vi "Configure TimersCounters UE9.vi"(0 "Handle In":i32, 1 "Enable Counter0":bool, 2 "Enable Counter1":bool, 5 "Timer Clock Base (0=750k, 1=48M)":i32, 7 "Timer Clock Divisor":i32, 9 "# Timers Enabled":i32, 11 "error in":errorcluster, 12 "TimerModes":u8[](array[numeric])=[0, 0, 0, 0, 0, 0], 13 "TimerValues":dbl[](array[numeric])=[0.0, 0.0, 0.0, 0.0, 0.0, 0.0] format="%.2f") -> (4 "Handle Out":i32, 15 "error out":errorcluster)   [LabVIEW 2021]
panel:
  # "Timer0\n\nTimer1\n\nTimer2\n\nTimer3\n\nTimer4\n\nTimer5"
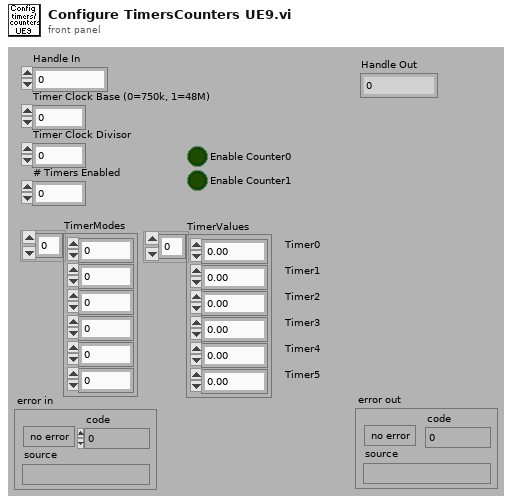
[diagram p1: front panel]
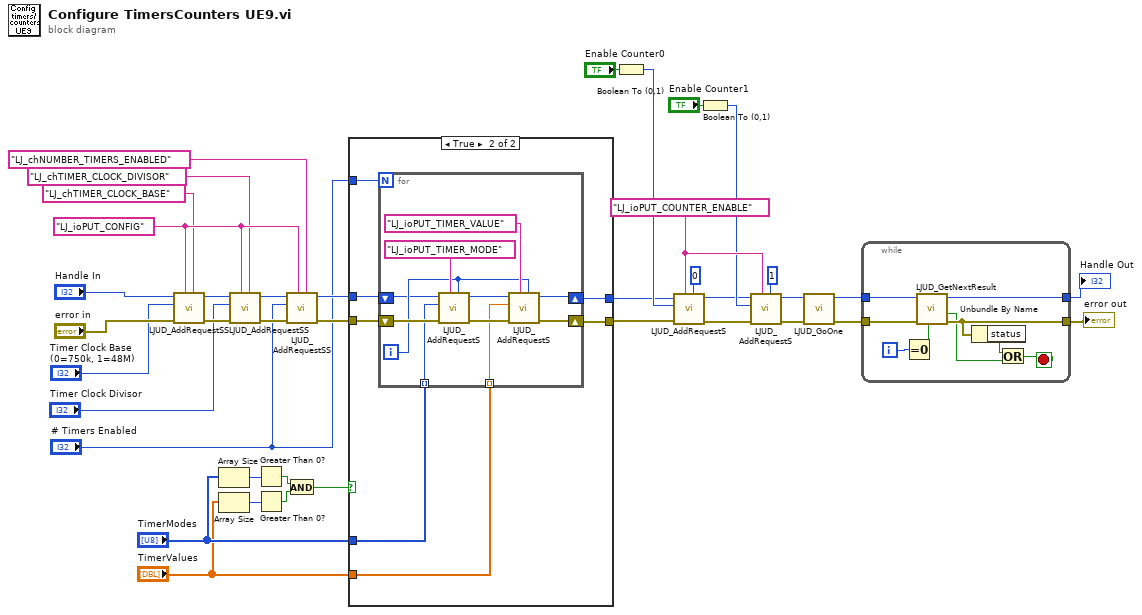
[diagram p0: block diagram]
diagram:
  w17 = "LJ_ioPUT_COUNTER_ENABLE" ("IOType")
  w35 = "LJ_ioPUT_CONFIG" ("IOType")
  n1 = call "LJUD_AddRequestSS.vi"("Channel"="LJ_chTIMER_CLOCK_BASE" ("IOType"), "IOType"=w35, "error in"="error in", "Value"="Timer Clock Base (0=750k, 1=48M)", "Handle In"="Handle In") -> ("error out"=w37:errorcluster, "Handle Out"=w39:i32)  [unwired: 5 in]
  n2 = Array Size(array="TimerModes") -> (size(s)=w22:i32)
  n3 = Array Size(array="TimerValues") -> (size(s)=w21:i32)
  n4 = call "LJUD_AddRequestSS.vi"("Channel"="LJ_chTIMER_CLOCK_DIVISOR" ("IOType"), "IOType"=w35, "error in"=w37, "Value"="Timer Clock Divisor", "Handle In"=w39) -> ("error out"=w36:errorcluster, "Handle Out"=w38:i32)  [unwired: 5 in]
  n5 = Greater Than 0?(x=w22) -> (x > 0?=w19:bool)
  n6 = Greater Than 0?(x=w21) -> (x > 0?=w20:bool)
  n7 = call "LJUD_AddRequestSS.vi"("Channel"="LJ_chNUMBER_TIMERS_ENABLED" ("IOType"), "IOType"=w35, "error in"=w36, "Value"="# Timers Enabled", "Handle In"=w38) -> ("error out"=w25:errorcluster, "Handle Out"=w10:i32)  [unwired: 5 in]
  n8 = And(x=w19, y=w20) -> (x .and. y?=w23:bool)
  n9 = case shown="True" w23 {
    tunnel: w25 -> [w41 w48]
    tunnel: "TimerModes" -> [_ w47]
    tunnel: "TimerValues" -> [_ w46]
    tunnel: [w41 w45] -> w18
    tunnel: w10 -> [w40 w44]
    tunnel: [w40 w43] -> w9
    tunnel: "# Timers Enabled" -> [_ w42]
    frame False {
    }
    frame True {
      n10 = for {
        N: w42 -> [_]
        shift-right: [w51] -> w45
        shift-left: w48 -> [w55]
        tunnel: w47 -> [w54] mode=indexing
        tunnel: w46 -> [w53] mode=indexing
        shift-right: [w49] -> w43
        shift-left: w44 -> [w50]
        i -> [w52]
        n11 = call "LJUD_AddRequestS.vi"("Channel"=w52, "IOType"="LJ_ioPUT_TIMER_MODE", "error in"=w55, "Value"=w54, "Handle In"=w50) -> ("error out"=w57:errorcluster, "Handle Out"=w56:i32)  [unwired: 5 in]
        n12 = call "LJUD_AddRequestS.vi"("Channel"=w52, "IOType"="LJ_ioPUT_TIMER_VALUE", "error in"=w57, "Value"=w53, "Handle In"=w56) -> ("error out"=w51:errorcluster, "Handle Out"=w49:i32)  [unwired: 5 in]
      }
    }
  }
  n13 = Boolean To (0,1)(Boolean="Enable Counter0") -> (0, 1=w14:i16)
  n14 = call "LJUD_AddRequestS.vi"("Channel"=0, "IOType"=w17, "error in"=w18, "Value"=w14, "Handle In"=w9) -> ("error out"=w12:errorcluster, "Handle Out"=w8:i32)  [unwired: 5 in]
  n15 = Boolean To (0,1)(Boolean="Enable Counter1") -> (0, 1=w13:i16)
  n16 = call "LJUD_AddRequestS.vi"("Channel"=1, "IOType"=w17, "error in"=w12, "Value"=w13, "Handle In"=w8) -> ("error out"=w11:errorcluster, "Handle Out"=w7:i32)  [unwired: 5 in]
  n17 = call "LJUD_GoOne.vi"("error in"=w11, "Handle In"=w7) -> ("error out"=w30:errorcluster, "Handle Out"=w31:i32)  [unwired: 8 in]
  n18 = while {
    tunnel: w30 -> [w66]
    tunnel: w31 -> [w65]
    tunnel: [w64] -> w6
    tunnel: [w62] -> w5
    i -> [w61]
    stop <- w68 stop-if-true
    n19 = Equal To 0?(x=w61) -> (x = 0?=w67:bool)
    n20 = call "LJUD_GetNextResult.vi"("GetFirst"=w67, "error in"=w66, "Handle In"=w65) -> ("error out"=w64:errorcluster, "LJE_NO_MORE_DATA_AVAILABLE"=w60:bool, "Handle Out"=w62:i32)  [unwired: 3 in, 3 out]
    n21 = Unbundle By Name(w64) -> ("status"=w63:bool)
    n22 = Or(x=w63, y=w60) -> (x .or. y?=w68:bool)
  }
  "error out" <- w6
  "Handle Out" <- w5
